vi "SetPort.vi"(8 "error in (no error)":errorcluster, 9 "Value":u8, 10 "Port":u8, 11 "MCU in":refnum<class "MCU.lvclass">) -> (0 "error out":errorcluster, 3 "MCU out":refnum<class "MCU.lvclass">)   [LabVIEW 2020, in "MCU.lvclass"]
doc: "Set a value on a port on the target device."
uses:
  MCU.lvclass
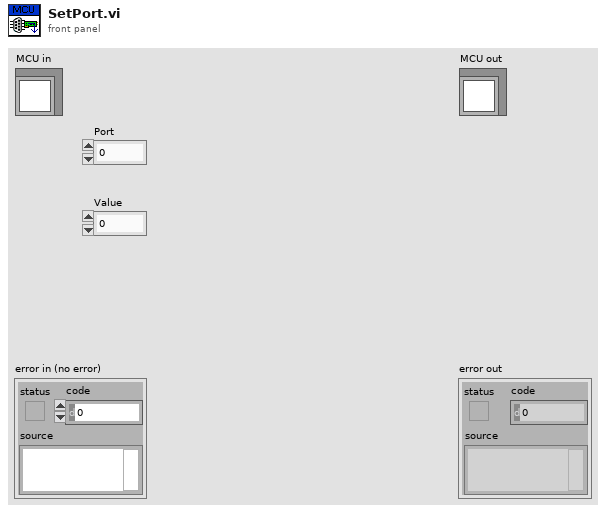
[diagram p1: front panel]
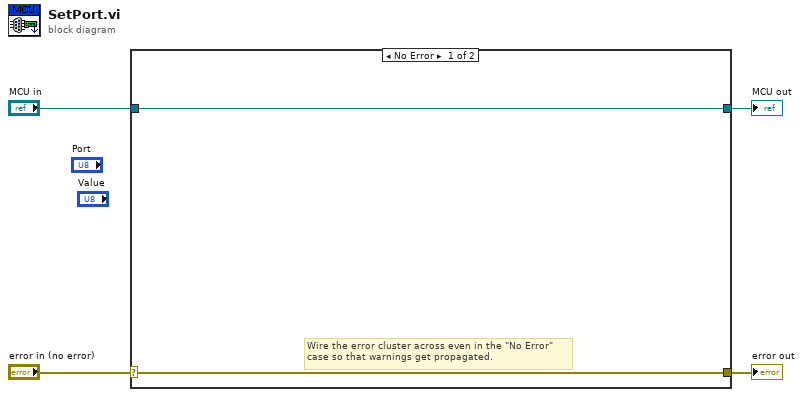
[diagram p0: block diagram]
diagram:
  n1 = case shown="No Error" "error in (no error)" {
    selector: "error in (no error)" -> [w5 w8]
    tunnel: [w5 w8] -> w3
    tunnel: [w6 w7] -> w1
    tunnel: "MCU in" -> [w6 w7]
    frame No Error {
      # "Wire the error cluster across even in the \"No Error\"\ncase so that warnings get propagated."
    }
    frame Error {
    }
  }
  "error out" <- w3
  "MCU out" <- w1
